vi "new detach communicator message.vi"(11 "communicator to detach":string) -> (3 "message":refnum<class "communicator message.lvclass">)   [LabVIEW 2015, in "queue manager.lvclass"]
uses:
  queue manager.lvclass
  message/communicator message.lvclass
  message/communicator message.lvclass/communicator message.ctl
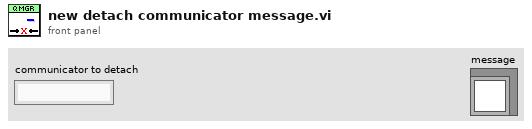
[diagram p1: front panel]
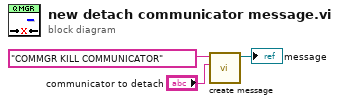
[diagram p0: block diagram]
diagram:
  n1 = call "create message.vi"("data"="communicator to detach", "ID"="COMMGR KILL COMMUNICATOR") -> ("message"=→"message":refnum<class "communicator message.lvclass">)  [unwired: 9 in]
